vi "registration.vi"(11 "client handle":T1) -> (3 "client handle out":T1)   [LabVIEW 2012]
uses:
  <vilib>/httpClient/ClientHandle.ctl
  <vilib>/httpClient/PUTBuffer.vi
  <vilib>/httpClient/LabVIEWHTTPClient.lvlib
panel:
  out "body":string
  out "Tasks URL":string
  out "Instructions URL":string
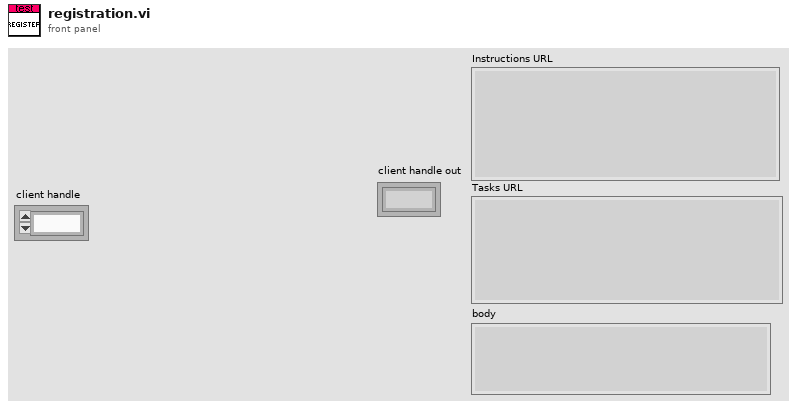
[diagram p1: front panel]
types:
  T1 = typedef "LabVIEWHTTPClient.lvlib/ClientHandle.ctl" = refnum<k1>
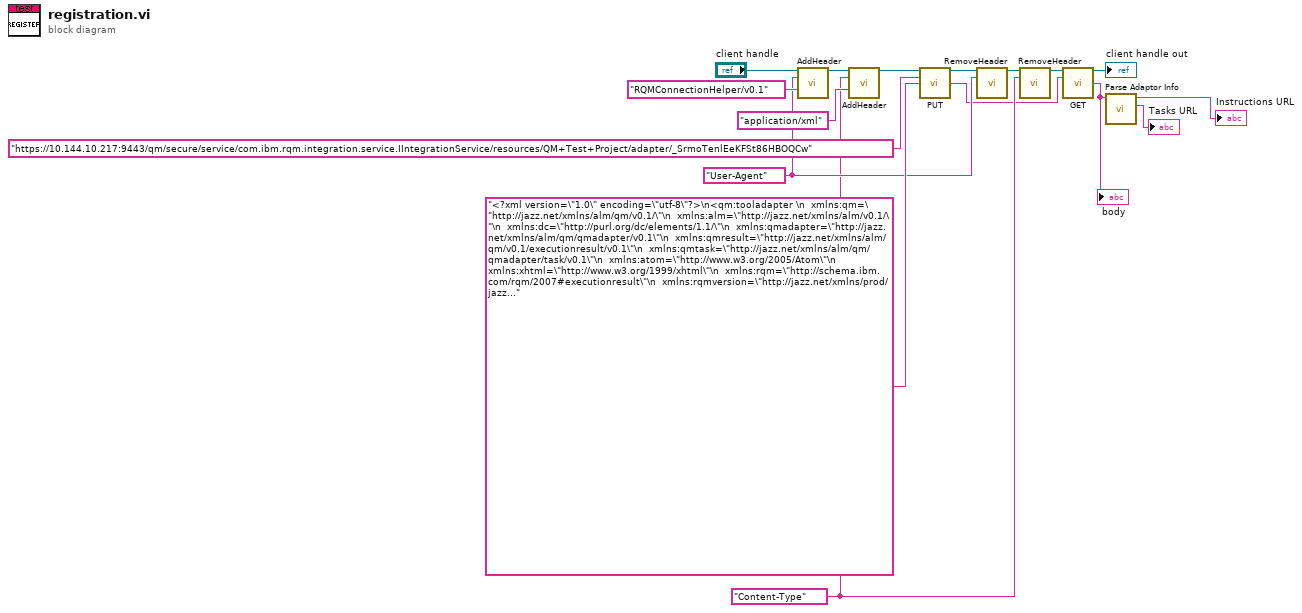
[diagram p0: block diagram]
diagram:
  w7 = "Content-Type" ("header")
  w8 = "User-Agent" ("header")
  n1 = call <vilib>:"AddHeader.vi"("client handle"="client handle", "header"=w8, "value"="RQMConnectionHelper/v0.1") -> ("client handle out"=w16:T1)  [unwired: 11 in, 1 out]
  n2 = call <vilib>:"AddHeader.vi"("client handle"=w16, "header"=w7, "value"="application/xml") -> ("client handle out"=w13:T1)  [unwired: 11 in, 1 out]
  n3 = call-poly <vilib>:"PUT.vi"("client handle"=w13, "url"="https://10.144.10.217:9443/qm/secure/service/com.ibm.rqm.integration.service.IIntegrationService/resources/QM+Test+Project/adapter/_SrmoTenlEeKFSt86HBOQCw", "buffer"="<?xml version=\"1.0\" encoding=\"utf-8\"?>\n<qm:tooladapter \n  xmlns:qm=\"http://jazz.net/xmlns/alm/qm/v0.1/\"\n  xmlns:alm=\"http://jazz.net/xmlns/alm/v0.1/\"\n  xmlns:dc=\"http://purl.org/dc/elements/1.1/\"\n  xmlns:qmadapter=\"http://jazz.net/xmlns/alm/qm/qmadapter/v0.1\"\n  xmlns:qmresult=\"http://jazz.net/xmlns/alm/qm/v0.1/executionresult/v0.1\"\n  xmlns:qmtask=\"http://jazz.net/xmlns/alm/qm/qmadapter/task/v0.1\"\n  xmlns:atom=\"http://www.w3.org/2005/Atom\"\n  xmlns:xhtml=\"http://www.w3.org/1999/xhtml\"\n  xmlns:rqm=\"http://schema.ibm.com/rqm/2007#executionresult\"\n  xmlns:rqmversion=\"http://jazz.net/xmlns/prod/jazz/rqm/qm/1.0/\"\n>\n<dc:identifier>_SrmoTenlEeKFSt86HBOQCw</dc:identifier>\n<dc:title>test</dc:title>\n<dc:description></dc:description>\n<dc:creator>test</dc:creator>\n<qmadapter:type>com.ni.rqm.adapter</qmadapter:type>\n<qmadapter:pollinginterval>0</qmadapter:pollinginterval>\n<qmadapter:state>AVAILABLE</qmadapter:state>\n<qmadapter:hostname>sh-rd-rwang</qmadapter:hostname>\n<qmadapter:ipaddress>10.144.8.51</qmadapter:ipaddress>\n<qmadapter:macaddress>00-FF-5D-B4-13-94</qmadapter:macaddress>\n<qmadapter:fqdn>sh-rd-rwang.apac.corp.natinst.com</qmadapter:fqdn>\n</qm:tooladapter>") -> ("client handle out"=w10:T1, "body"=w5:string)  [unwired: 9 in, 2 out]
  n4 = call <vilib>:"RemoveHeader.vi"("client handle"=w10, "header"=w8) -> ("client handle out"=w9:T1)  [unwired: 12 in, 1 out]
  n5 = call <vilib>:"RemoveHeader.vi"("client handle"=w9, "header"=w7) -> ("client handle out"=w6:T1)  [unwired: 12 in, 1 out]
  n6 = call <vilib>:"GET.vi"("client handle"=w6, "url"=w5) -> ("client handle out"=→"client handle out":T1, "body"=w4:string)  [unwired: 10 in, 2 out]
  "body" <- w4
  n7 = call "Parse Adaptor Info.vi"("Adaptor Info XML"=w4) -> ("Tasks URL"=→"Tasks URL":string, "Instructions URL"=→"Instructions URL":string)  [unwired: 8 in, 1 out]
